vi "Lesson 2-2 Filtering the Signal.vi"() -> ()   [LabVIEW 2020]
uses:
  Lesson 1/HRM-AQN-input_clust.ctl
panel:
  in  "Additional Signal to remove [s]":i32
  out "Filtered data":waveform(dbl)(graph)
  in  "samples [s]":i32
  out "Raw collected data":waveform(dbl)(graph)
  out "error out":errorcluster
  in  "stop":bool
  out "Raw data":waveform(dbl)(graph)
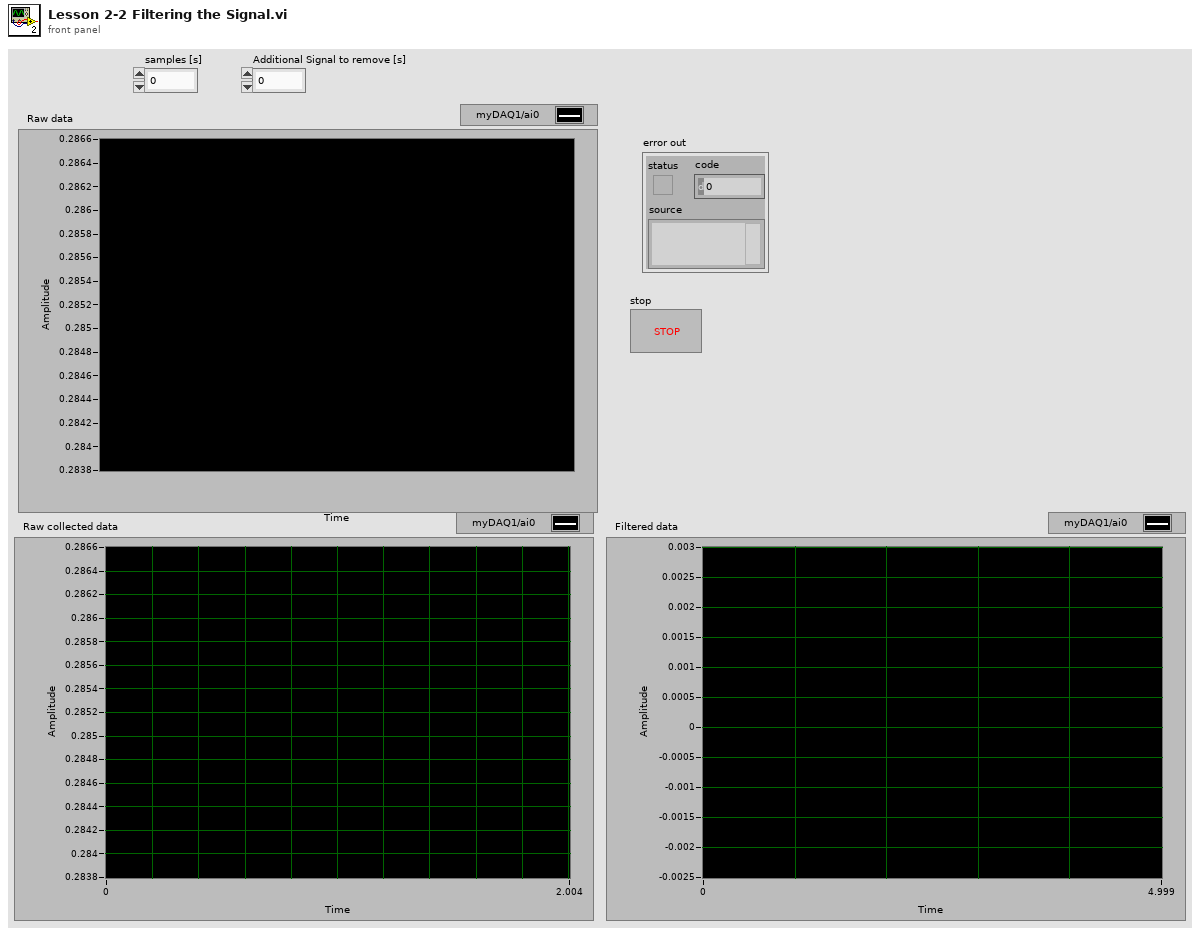
[diagram p1: front panel]
types:
  T1 = typedef "HRM-AQN-input_clust.ctl" = cluster{"physical channels":tag, "myDAQ task":refnum<k21>}
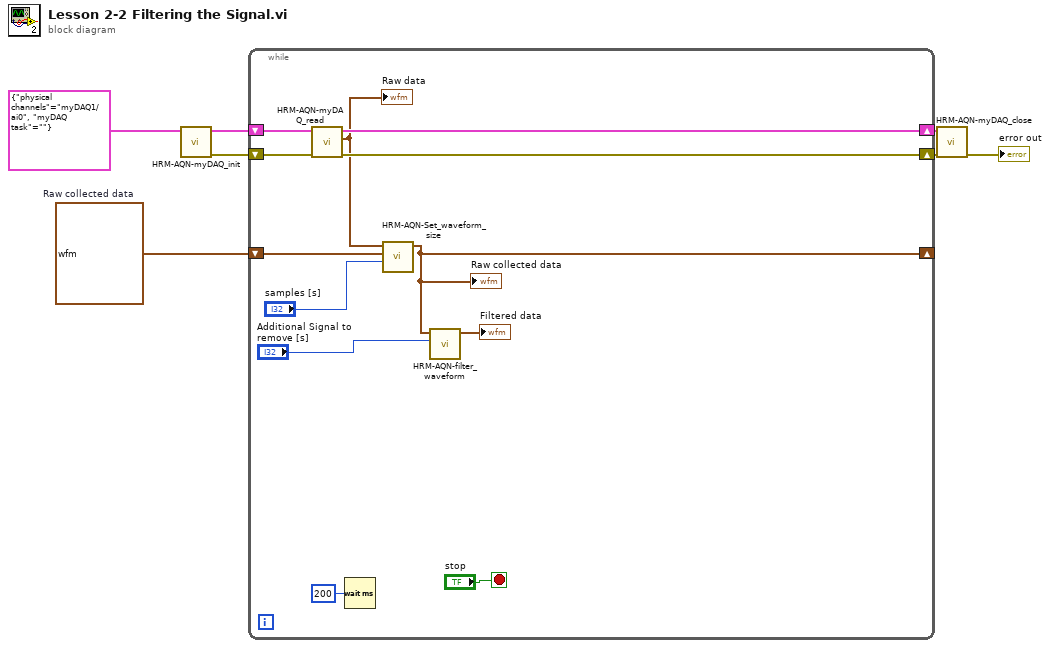
[diagram p0: block diagram]
diagram:
  w1 = waveform(dbl) {"t0"=timestamp(0 s since 1904-01-01), "dt"=1.0, "Y"=[]}  # Raw collected data
  n1 = call "HRM-AQN-myDAQ_init.vi"("AQN cluster in"=T1 {"physical channels"="myDAQ1/ai0", "myDAQ task"=""}) -> ("error out"=w7:errorcluster, "AQN cluster out"=w3:T1)  [unwired: 9 in]
  n2 = while {
    shift-right: [w14] -> w2
    shift-left: w3 -> [w15]
    shift-right: [w18] -> w6
    shift-left: w7 -> [w19]
    shift-right: [w10] -> _
    shift-left: w1 -> [w13]
    stop <- "stop" stop-if-true
    n3 = call "HRM-AQN-myDAQ_read.vi"("error in (no error)"=w19, "AQN cluster in"=w15) -> ("error out"=w18:errorcluster, "data"=w12:waveform(dbl), "AQN cluster out"=w14:T1)  [unwired: 7 in]
    "Raw data" <- w12
    n4 = Wait (ms)(milliseconds to wait=u32 200) -> ()  [unwired: 1 out]
    n5 = call "HRM-AQN-Set_waveform_size.vi"("samples [s]"="samples [s]", "Raw collected data"=w13, "data in"=w12) -> ("data out"=w10:waveform(dbl))  [unwired: 8 in]
    "Raw collected data" <- w10
    n6 = call "HRM-AQN-filter_waveform.vi"("Additional Signal to remove [s]"="Additional Signal to remove [s]", "data in"=w10) -> ("data out"=→"Filtered data":waveform(dbl))  [unwired: 9 in]
  }
  n7 = call "HRM-AQN-myDAQ_close.vi"("error in (no error)"=w6, "AQN cluster in"=w2) -> ("error out"=→"error out":errorcluster)  [unwired: 9 in]
